vi "Save String Array.vi"(7 "section":string, 8 "error in (no error)":errorcluster, 9 "String Array In":string[](array[string]), 10 "key":string, 11 "refnum":T1) -> (0 "error out":errorcluster, 3 "refnum out":T1)   [LabVIEW 2013]
uses:
  <vilib>/Utility/config.llb/Config Data RefNum.ctl
  <vilib>/Utility/config.llb/Write Key (String).vi
  <vilib>/Utility/config.llb/NI_LVConfig.lvlib
panel:
  out "Joined Result":string
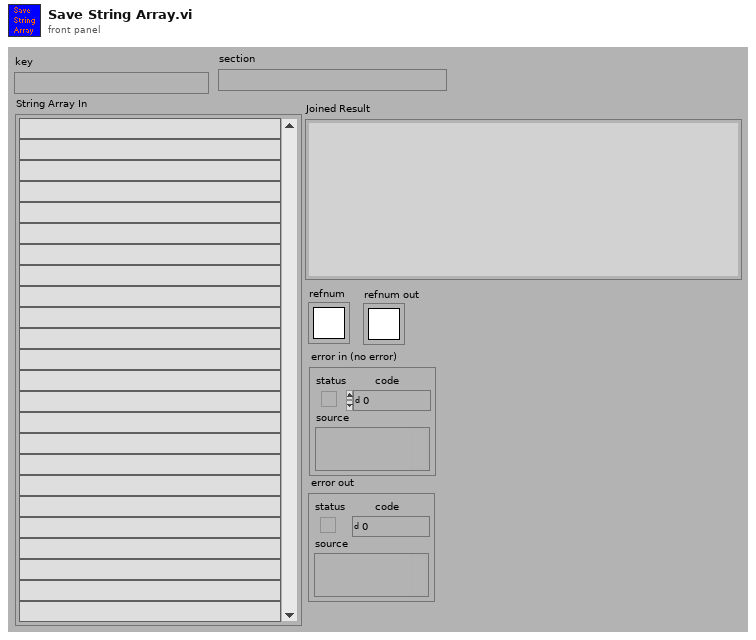
[diagram p1: front panel]
types:
  T1 = typedef "NI_LVConfig.lvlib/Config Data RefNum.ctl" = refnum<k1>
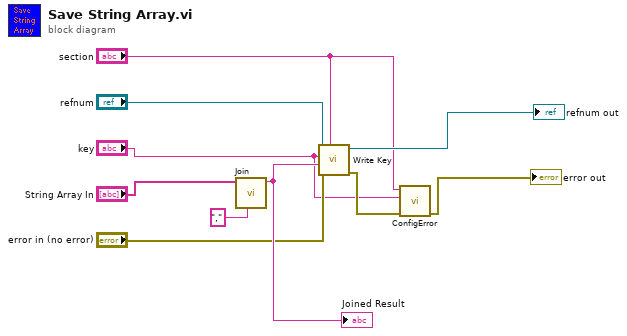
[diagram p0: block diagram]
diagram:
  n1 = call "Join.vi"("delimiter"=",", "Array"="String Array In") -> ("Joined Result"=w8:string)  [unwired: 9 out]
  "Joined Result" <- w8
  n2 = call-poly <vilib>:"Write Key.vi"("section"="section", "error in (no error)"="error in (no error)", "value"=w8, "key"="key", "refnum"="refnum") -> ("error out"=w4:errorcluster, "refnum out"=→"refnum out":T1)  [unwired: 1 in, 4 out]
  n3 = call "ConfigError.vi"("error in (no error)"=w4, "Key"="key", "Section"="section") -> ("error out"=→"error out":errorcluster)  [unwired: 8 out]
